vi "MPExxx_Sett_example.vi"() -> ()   [LabVIEW 2012]
doc: "This VI form sets all the set points for the current memory location."
panel:
  out "error out":errorcluster
  in  "error in (no error)":errorcluster
  in  "OCP":dbl format="%.2f"
  in  "OVP":dbl format="%.2f"
  in  "Current":dbl format="%.2f"
  in  "Voltage":dbl format="%.2f"
  in  "VISA Resource Name":refnum<visa-resource-name>
  # "MAGNA-POWER"
  # "Electronics"
  # "Instrument Settings"
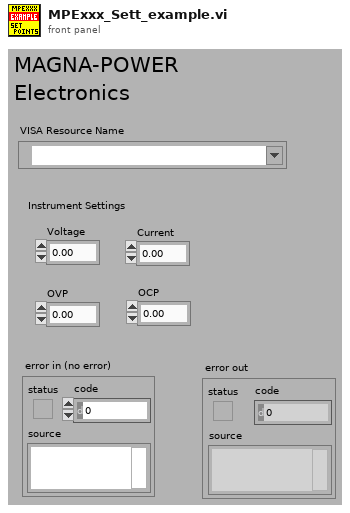
[diagram p1: front panel]
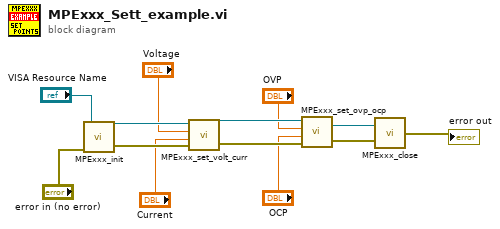
[diagram p0: block diagram]
diagram:
  n1 = call "MPExxx_init.vi"("error in (no error)"="error in (no error)", "VISA session"="VISA Resource Name") -> ("error out"=w12:errorcluster, "dup VISA session"=w9:refnum<visa-resource-name>)  [unwired: 2 in]
  n2 = call "MPExxx_set_volt_curr.vi"("error in (no error)"=w12, "Set Current"="Current", "Set Voltage"="Voltage", "VISA session"=w9) -> ("error out"=w11:errorcluster, "dup VISA session"=w10:refnum<visa-resource-name>)
  n3 = call "MPExxx_set_ovp_ocp.vi"("error in (no error)"=w11, "Set OCP"="OCP", "Set OVP"="OVP", "VISA session"=w10) -> ("error out"=w2:errorcluster, "dup VISA session"=w1:refnum<visa-resource-name>)
  n4 = call "MPExxx_close.vi"("error in (no error)"=w2, "VISA session"=w1) -> ("error out"=→"error out":errorcluster)
